vi "Read Measurement Data.vi"(7 "Data Size (0)":i32, 8 "error in (no error)":errorcluster, 9 "Data Offset (0)":i32, 10 "Channel (1: Channel 1)":i32(ring)=1 items=["Channel 1"=1, "Channel 2"=2], 11 "VISA resource name":refnum<visa-resource-name>) -> (0 "error out":errorcluster, 2 "Measurement Data":dbl[](array[numeric]), 3 "VISA resource name out":refnum<visa-resource-name>)   [LabVIEW 2012, in "Keysight B2980 Series.lvlib"]
doc: "Returns the array data which contains all of the current measurement data, voltage measurement data, resistance measurement data, source output setting data, status data, or time data."
uses:
  Keysight B2980 Series.lvlib
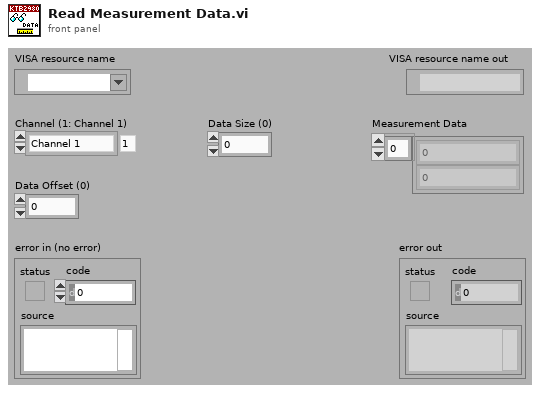
[diagram p1: front panel]
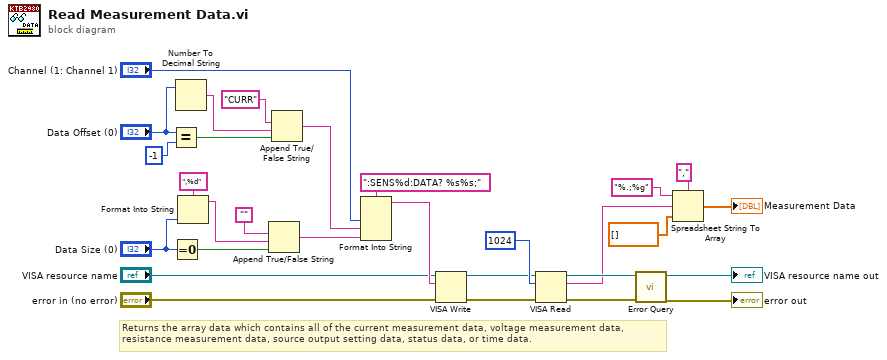
[diagram p0: block diagram]
diagram:
  # "Returns the array data which contains all of the current measurement data, voltage measurement data, \nresistance measurement data, source output setting data, status data, or time data."
  n1 = Equal?(x="Data Offset (0)", y=-1) -> (x = y?=w10:bool)
  n2 = Equal To 0?(x="Data Size (0)") -> (x = 0?=w6:bool)
  n3 = Number To Decimal String(number="Data Offset (0)") -> (decimal integer string=w8:string)  [unwired: 1 out]
  n4 = Format Into String(format string=",%d", "Data Size (0)") -> (resulting string=w3:string)  [unwired: 2 in, 1 out]
  n5 = Append True/False String(1:w6, 2:w3, 3:"") -> (0:w4:string)  [unwired: 1 in]
  n6 = Append True/False String(1:w10, 2:w8, 3:"CURR") -> (0:w7:string)  [unwired: 1 in]
  n7 = Format Into String(format string=":SENS%d:DATA? %s%s;", "Channel (1: Channel 1)", w7, w4) -> (resulting string=w28:string)  [unwired: 2 in, 1 out]
  n8 = VISA Write(VISA resource name="VISA resource name", write buffer=w28, error in (no error)="error in (no error)") -> (VISA resource name out=w24:refnum<visa-resource-name>, error out=w23:errorcluster)  [unwired: 1 out]
  n9 = VISA Read(VISA resource name=w24, byte count=u32 1024, error in (no error)=w23) -> (VISA resource name out=w22:refnum<visa-resource-name>, read buffer=w15:string, error out=w21:errorcluster)  [unwired: 1 out]
  n10 = call "Error Query.vi"("error in (no error)"=w21, "VISA resource name"=w22) -> ("error out"=→"error out":errorcluster, "VISA resource name out"=→"VISA resource name out":refnum<visa-resource-name>)  [unwired: 8 out]
  n11 = Spreadsheet String To Array(delimiter (Tab)=",", format string="%.;%g", spreadsheet string=w15, array type (2D Dbl)=dbl[] []) -> (array=→"Measurement Data":dbl[])
